vi "HT_Contents_GUI.vi"   [LabVIEW 2014]
doc: "This \"contents\" VI contains all components of CS, which are specific for YOU, a CS user. Add your own stuff here."
uses:
  HitrapGUI/HitrapGUI.lvlib
  CSGui/GOGControllerGUI/GOGControllerGUI.lvlib
  Hitrap_DiagnosticBoxGUI/Hitrap_DiagnosticBoxGUI.lvlib
  CSGui/ISEG_HVBoardGUI/ISEG_HVBoardGUI.lvlib
  CSGui/ISEG_HVSystemGUI/ISEG_HVSystemGUI.lvlib
  CSConnectGUI/CSConnectGUI.lvlib
  CSGui/IMAQController/IMAQController.lvlib
  CSPentatrap/PTScanner/PTScanner.lvlib
  CSPentatrap/PTSequencer/PTSequencer.lvlib
  CSGui/PPG_ABCGUI/PPG_ABCGUI.lvlib
  CSGui/KE6485GUI/KE6485GUI.lvlib
  CSDigitalIO/DIM_DIO/DIM_DIO.lvlib
  HTVacuum/HTVacuum.lvlib
  HTVacuumGUI/HTVacuumGUI.lvlib
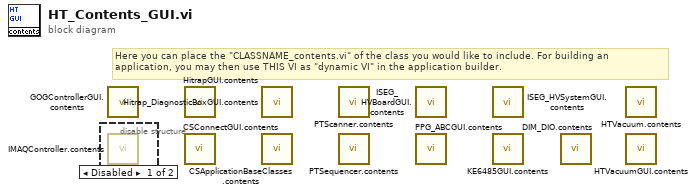
[diagram p0: block diagram]
diagram:
  # "Here you can place the \"CLASSNAME_contents.vi\" of the class you would like to include. For building an \napplication, you may then use THIS VI as \"dynamic VI\" in the application builder."
  n1 = disable-structure shown="Disabled" {
    frame Disabled {
      n2 = call "IMAQController.contents.vi"() -> ()  [unwired: 1 in]
    }
    frame Enabled {
    }
  }
  n3 = call "GOGControllerGUI.contents.vi"() -> ()  [unwired: 1 in]
  n4 = call "HitrapGUI.contents.vi"() -> ()  [unwired: 1 in]
  n5 = call "CSConnectGUI.contents.vi"() -> ()  [unwired: 1 in]
  n6 = call "Hitrap_DiagnosticBoxGUI.contents.vi"() -> ()  [unwired: 1 in]
  n7 = call "CSApplicationBaseClasses.contents.vi"() -> ()  [unwired: 1 in]
  n8 = call "PTScanner.contents.vi"() -> ()  [unwired: 1 in]
  n9 = call "PTSequencer.contents.vi"() -> ()  [unwired: 1 in]
  n10 = call "ISEG_HVBoardGUI.contents.vi"() -> ()  [unwired: 1 in]
  n11 = call "PPG_ABCGUI.contents.vi"() -> ()  [unwired: 1 in]
  n12 = call "ISEG_HVSystemGUI.contents.vi"() -> ()  [unwired: 1 in]
  n13 = call "KE6485GUI.contents.vi"() -> ()  [unwired: 20 in]
  n14 = call "DIM_DIO.contents.vi"() -> ()  [unwired: 1 in]
  n15 = call "HTVacuum.contents.vi"() -> ()  [unwired: 20 in]
  n16 = call "HTVacuumGUI.contents.vi"() -> ()  [unwired: 20 in]
